vi "Begin.vi"() -> (0 "error out":errorcluster)   [LabVIEW 2013]
doc: "Called before other user functions, this VI is expected to open initial I/O refnums, load in file data, and do all program initialization. Notice that the <B>error out</B> terminal is simply used for data flow. Wiring it to other structures or subVIs ensures that this VI runs first."
uses:
  <vilib>/Rock Robotics/WPI/DriverStation/WPI_DriverStationRobotMode2.ctl
  <vilib>/Rock Robotics/WPI/Joystick/WPI_JoystickDeviceEnum.ctl
  <vilib>/Rock Robotics/SystemInterfaces/DIO/FPGA_DIORelayChannel.ctl
  <vilib>/Rock Robotics/SystemInterfaces/DIO/FPGA_DIOChannel.ctl
  <vilib>/Rock Robotics/SystemInterfaces/Typedef/FPGA_TypedefDigitalModule.ctl
  <vilib>/Rock Robotics/WPI/Solenoid/WPI_SolenoidChannel.ctl
  <vilib>/Rock Robotics/SystemInterfaces/DIO/FPGA_DIOPWMChannel.ctl
  <vilib>/Rock Robotics/WPI/SafetyOutput/WPI_SafetyOutputConfigMenu.ctl
  TankDriveAction.ctl
  PnuematicMode.ctl
  <vilib>/Rock Robotics/WPI/Camera/WPI_CameraWhite Balance Values.ctl
  <vilib>/Rock Robotics/WPI/Camera/WPI_CameraExposure Values.ctl
  <vilib>/Rock Robotics/WPI/Camera/WPI_CameraFrameRate.ctl
  <vilib>/Rock Robotics/WPI/Camera/WPI_CameraImageSize.ctl
  OccurrenceAction.ctl
  NotifierAction.ctl
  Example_Code/Gyro/Read Angle Mode.ctl
  <vilib>/Rock Robotics/SystemInterfaces/Typedef/FPGA_TypedefAnalogModuleForGyro.ctl
  <vilib>/Rock Robotics/SystemInterfaces/AI/FPGA_AIGyroChannel.ctl
  Robot Global Data.vi
  <vilib>/Rock Robotics/WPI/Solenoid/WPI_SolenoidOpenSingle.vi
  <vilib>/Rock Robotics/WPI/RobotDrive/WPI_RobotDriveOpen4MotorWithTalon.vi
  ErrorTest/OutputError.vi
  <vilib>/Rock Robotics/WPI/Compressor/WPI_CompressorGetSetRefNum.vi
  <vilib>/Rock Robotics/WPI/Counter/WPI_CounterDigitalInputToDigitalSource.vi
  <vilib>/Rock Robotics/WPI/Encoder/WPI_EncoderType.ctl
panel:
  in  "Gain (VoltsPerDegree/Second)":dbl=0.007
  in  "Version":string="1.3.1"
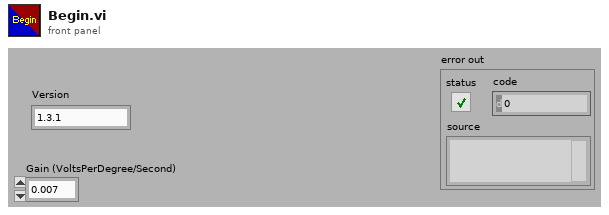
[diagram p1: front panel]
types:
  T1 = typedef "FPGA_AIGyroChannel.ctl" = enum8{"AI 1", "AI 2", "Invalid"}
  T2 = typedef "FPGA_TypedefAnalogModuleForGyro.ctl" = enum16{"Analog Module 1"}
  T3 = typedef "Read Angle Mode.ctl" = enum16{"Init", "ReadAngle", "Disable"}
  T4 = typedef "NotifierAction.ctl" = enum16{"Init", "Get"}
  T5 = typedef "OccurrenceAction.ctl" = enum16{"Init", "Get", "Set"}
  T6 = typedef "WPI_CameraImageSize.ctl" = enum16{"640x480", "320x240", "160x120"}
  T7 = typedef "WPI_CameraFrameRate.ctl" = u32
  T8 = typedef "WPI_CameraExposure Values.ctl" = enum16{"Auto", "Flicker-free 50 Hz", "Flicker-free 60 Hz", "Hold current"}
  T9 = typedef "WPI_CameraWhite Balance Values.ctl" = enum16{"Auto", "Fixed indoor", "Fixed outdoor 1", "Fixed outdoor 2", "Fixed fluorescent 1", "Fixed fluorescent 2", "Hold current"}
  T10 = typedef "PnuematicMode.ctl" = enum16{"Init", "SetState", "Disable"}
  T11 = typedef "WPI_SolenoidChannel.ctl" = enum8{"Solenoid 1", "Solenoid 2", "Solenoid 3", "Solenoid 4", "Solenoid 5", "Solenoid 6", "Solenoid 7", "Solenoid 8", "Invalid"}
  T12 = typedef "FPGA_DIOPWMChannel.ctl" = enum8{"PWM 1", "PWM 2", "PWM 3", "PWM 4", "PWM 5", "PWM 6", "PWM 7", "PWM 8", "PWM 9", "PWM 10", "Invalid"}
  T13 = typedef "TankDriveAction.ctl" = enum16{"Init", "LinearDrive", "SetValue", "Disable"}
  T14 = typedef "WPI_SafetyOutputConfigMenu.ctl" = enum16{"Enable", "Disable"}
  T15 = typedef "FPGA_TypedefDigitalModule.ctl" = enum16{"Digital Module 1", "Digital Module 2"}
  T16 = typedef "FPGA_DIOChannel.ctl" = enum8{"DIO 1", "DIO 2", "DIO 3", "DIO 4", "DIO 5", "DIO 6", "DIO 7", "DIO 8", "DIO 9", "DIO 10", "DIO 11", "DIO 12", "DIO 13", "DIO 14", "Invalid"}
  T17 = typedef "FPGA_DIORelayChannel.ctl" = enum8{"Relay 1", "Relay 2", "Relay 3", "Relay 4", "Relay 5", "Relay 6", "Relay 7", "Relay 8", "Invalid"}
  T18 = typedef "WPI_JoystickDeviceEnum.ctl" = enum16{"USB 1", "USB 2", "USB 3", "USB 4", "Kinect 1", "Kinect 2"}
  T19 = typedef "WPI_DriverStationRobotMode2.ctl" = enum16{"Autonomous Disabled", "Autonomous Enabled", "Teleop Disabled", "Teleop Enabled", "Timeout", "Finish", "Test Disabled", "Test Enabled"}
  T20 = typedef "WPI_EncoderType.ctl" = enum16{"1x", "2x", "4x"}
  T21 = typedef "WPI_DigitalInputDevRef.ctl" = cluster{"DevStatus":errorcluster, "DIO Channel":T16, "Digital Module":T15}
  T22 = typedef "FPGA_CounterEncoderSourceConvertionLVSourceType.ctl" = cluster{"DevStatus":errorcluster, "AnalogTriggerMode?":bool, "DigitalMode":cluster{"Digital Module":T15, "DIO Channel":T23}, "AnalogTriggerMode":cluster{"AnalogTriggerIndex":T24, "OutputType":T25}}
  T23 = typedef "FPGA_DIODigitalSourceChannel.ctl" = enum8{"DIO 1", "DIO 2", "DIO 3", "DIO 4", "DIO 5", "DIO 6", "DIO 7", "DIO 8", "DIO 9", "DIO 10", "DIO 11", "DIO 12", "DIO 13", "DIO 14", "Disabled"}
  T24 = typedef "FPGA_AnalogTriggerIndex.ctl" = enum8{"Trig 0", "Trig 1", "Trig 2", "Trig 3", "Trig 4", "Trig 5", "Trig 6", "Trig 7", "Invalid"}
  T25 = typedef "FPGA_AnalogTriggerOutType.ctl" = enum16{"InWindow", "TriggerState", "Rising", "Falling"}
  T26 = typedef "WPI_EncoderDevRef.ctl" = cluster{"DevStatus":errorcluster, "EncoderIndex":T27, "CounterIndex":T28, "DistancePerCount":dbl, "Decoding Type":T20}
  T27 = typedef "FPGA_EncoderIdx.ctl" = enum8{"Enc 0", "Enc 1", "Enc 2", "Enc 3", "Invalid"}
  T28 = typedef "FPGA_CounterCtrSystemIndex.ctl" = enum8{"Ctr 0", "Ctr 1", "Ctr 2", "Ctr 3", "Ctr 4", "Ctr 5", "Ctr 6", "Ctr 7", "Invalid"}
  T29 = typedef "WPI_SolenoidDevRef.ctl" = cluster{"DevStatus":errorcluster, "Solenoid Module":T30, "Forward Solenoid Channel":T11, "Reverse Solenoid Channel":T11}
  T30 = typedef "FPGA_TypedefSolenoidModule.ctl" = enum16{"Solenoid Module 1", "Solenoid Module 2"}
  T31 = typedef "WPI_RobotDriveDevRef.ctl" = cluster{"DevStatus":errorcluster, "Motors[]":T32[], "Square Inputs":bool, "Max Output":dbl, "Isochronous":bool}
  T32 = typedef "WPI_MotorControlDeviceRef.ctl" = cluster{"DeviceStatus":errorcluster, "Type":enum16{"PWM", "CAN"}, "PWM":cluster{"Digital Module":T15, "PWM Channel":T12, "DeadBand":T33}, "CAN":cluster{"Device Number":u8, "Control Mode":T34, "Semaphore":T35, "Max Vout":dbl}, "Invert":bool, "TransformRef":T36, "InvTransformRef":T36}
  T33 = typedef "WPI_PWMDeadband.ctl" = cluster{"Name":string, "maxPositivePwm":i32, "minPositivePwm":i32, "centerPwm":i32, "maxNegativePwm":i32, "minNegativePwm":i32, "angularRange":u16}
  T34 = typedef "WPI_CANJaguar_ControlMode.ctl" = enum8{"Percent VBus", "Current", "Speed", "Position", "Voltage"}
  T35 = typedef "Semaphore RefNum" = refnum<k1>
  T36 = typedef "WPI_PWMTransform_ConPane.ctl" = refnum<vi>
  T37 = typedef "WPI_CameraDevRef.ctl" = cluster{"Camera Address":string, "CameraStatus":errorcluster, "Acquire Image Notifier":refnum<notifier>}
  T38 = typedef "WPI_JoystickDevRef.ctl" = cluster{"Device":T18}
  T39 = typedef "WPI_CompressorDevRef.ctl" = cluster{"DevStatus":errorcluster, "DigitalInputDevRef":T21, "RelayDevRef":T40}
  T40 = typedef "WPI_RelayDevRef.ctl" = cluster{"DevStatus":errorcluster, "Relay Channel":T17, "Digital Module":T15, "Relay Direction":T41}
  T41 = typedef "WPI_RelayDirection.ctl" = enum16{"Both directions", "Forward only", "Reverse only"}
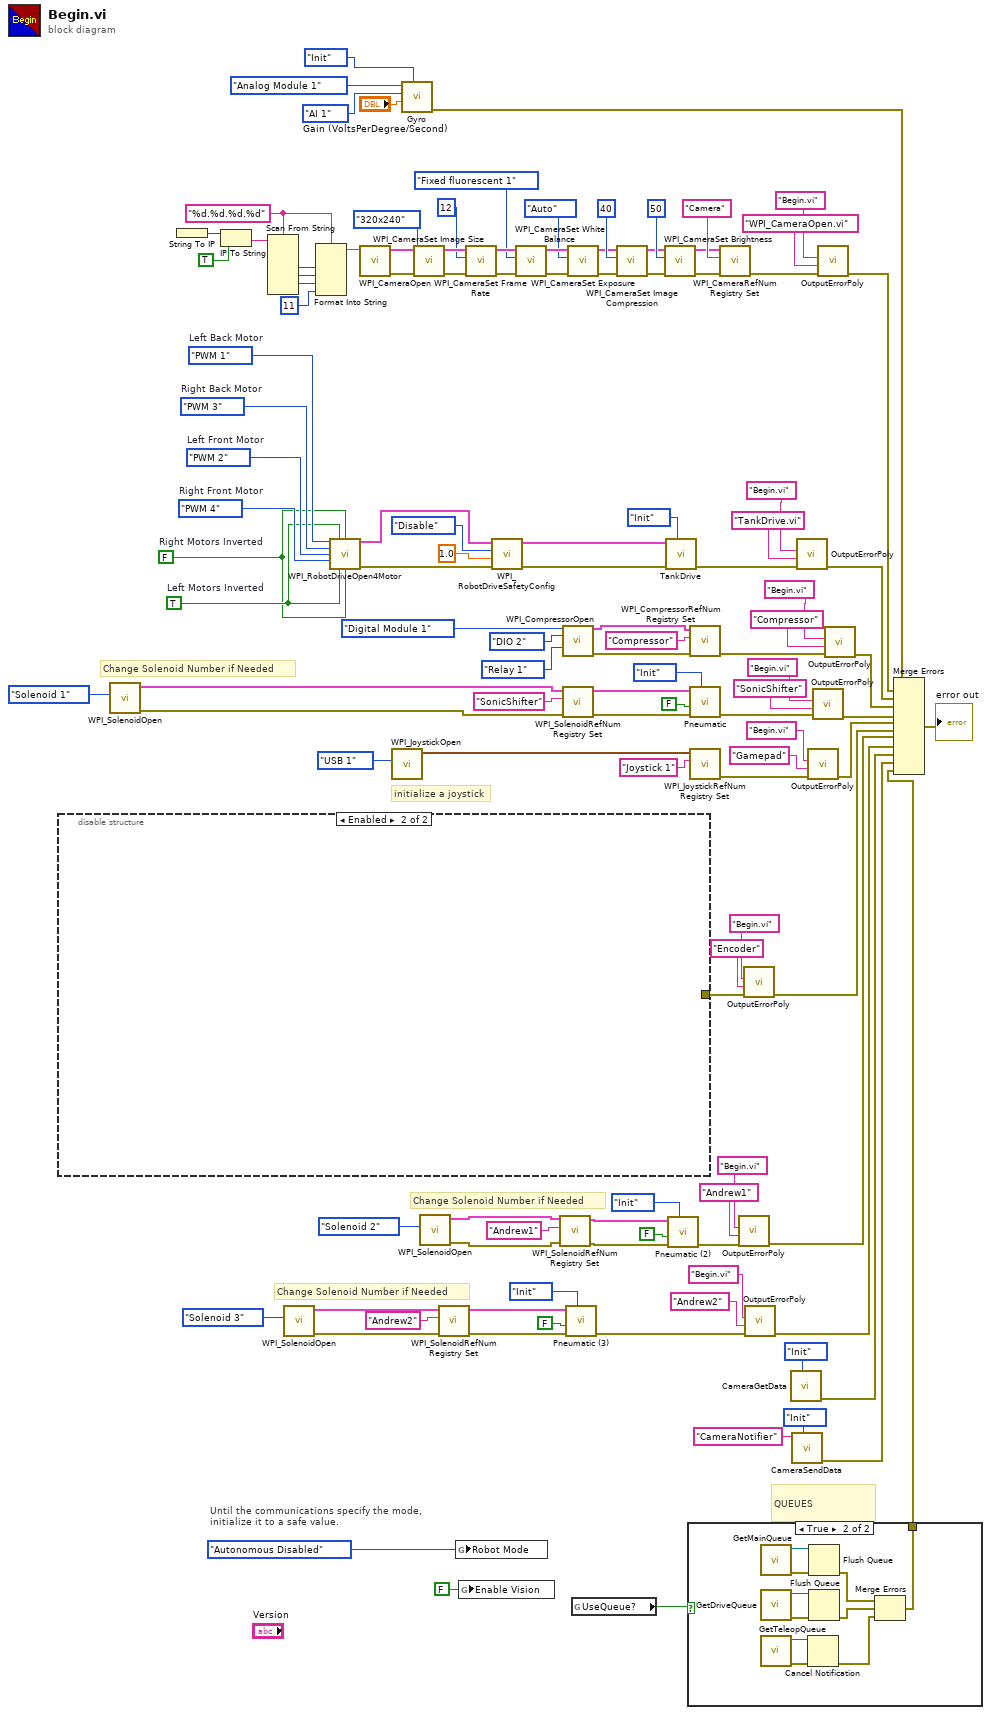
[diagram p0: block diagram]
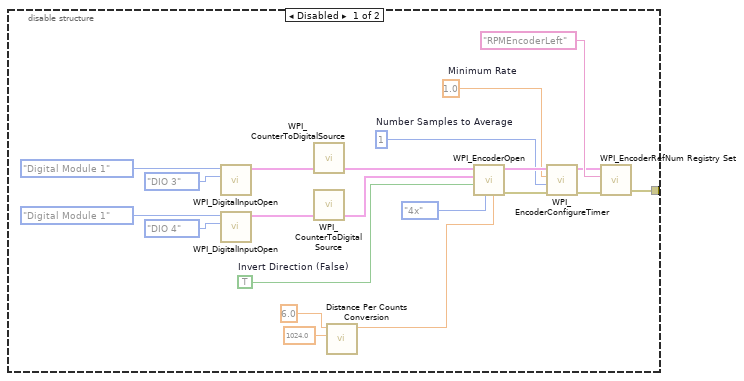
[diagram p3: hidden frame]
diagram:
  w51 = "%d.%d.%d.%d" ("format string")
  w103 = FPGA_DIOPWMChannel."PWM 4"  # Right Front Motor
  w104 = FPGA_DIOPWMChannel."PWM 2"  # Left Front Motor
  w109 = FPGA_DIOPWMChannel."PWM 3"  # Right Back Motor
  w110 = FPGA_DIOPWMChannel."PWM 1"  # Left Back Motor
  w101 = FALSE  # Right Motors Inverted
  w102 = TRUE  # Left Motors Inverted
  # "QUEUES"
  # "Change Solenoid Number if Needed"
  # "Change Solenoid Number if Needed"
  # "Change Solenoid Number if Needed"
  # "initialize a joystick"
  # "Until the communications specify the mode,\ninitialize it to a safe value."
  n1 = disable-structure shown="Enabled" {
    disable-tunnel: [w124 _] -> w33
    frame Disabled {
      w131 = TRUE  # Invert Direction (False)
      w133 = u8 1  # Number Samples to Average
      w134 = 1.0  # Minimum Rate
      n2 = call <vilib>:"WPI_DigitalInputOpen.vi"("DIO Channel"=FPGA_DIOChannel."DIO 3", "Digital Module (Module 1)"=FPGA_TypedefDigitalModule."Digital Module 1") -> ("DigitalInputDevRef"=w141:T21)  [unwired: 1 in, 8 out]
      n3 = call <vilib>:"WPI_DigitalInputOpen.vi"("DIO Channel"=FPGA_DIOChannel."DIO 4", "Digital Module (Module 1)"=FPGA_TypedefDigitalModule."Digital Module 1") -> ("DigitalInputDevRef"=w142:T21)  [unwired: 1 in, 8 out]
      n4 = call-poly <vilib>:"WPI_CounterToDigitalSource.vi"("DigitalInputDevRef"=w141) -> ("Digital Source"=w140:T22)  [unwired: 6 out]
      n5 = call-poly <vilib>:"WPI_CounterToDigitalSource.vi"("DigitalInputDevRef"=w142) -> ("Digital Source"=w143:T22)  [unwired: 6 out]
      n6 = call "Distance Per Counts Conversion.vi"("Counts Per Rev"=1024.0, "WheelDiameter"=6.0) -> ("Distance/Count"=w127:dbl)  [unwired: 9 in]
      n7 = call <vilib>:"WPI_EncoderOpen.vi"("DistancePerCount"=w127, "Decoding Type"=WPI_EncoderType."4x", "Invert Direction (False)"=w131, "BSource"=w143, "ASource"=w140) -> ("error out"=w129:errorcluster, "EncoderDevRef"=w137:T26)  [unwired: 3 in, 2 out]
      n8 = call <vilib>:"WPI_EncoderConfigureTimer.vi"("error in (no error)"=w129, "Number Samples to Average"=w133, "Minimum Rate"=w134, "EncoderDevRef"=w137) -> ("error out"=w128:errorcluster, "EncoderDevRef"=w130:T26)  [unwired: 6 out]
      n9 = call <vilib>:"WPI_EncoderRefNum Registry Set.vi"("error in (no error)"=w128, "refnum name"="RPMEncoderLeft", "EncoderDevRef"=w130) -> ("error out"=w124:errorcluster)  [unwired: 7 in, 1 out]
    }
    frame Enabled {
    }
  }
  n10 = call-poly <vilib>:"WPI_SolenoidOpen.vi"("Solenoid Channel"=WPI_SolenoidChannel."Solenoid 1") -> ("error out"=w111:errorcluster, "SolenoidDevRef"=w113:T29)  [unwired: 9 in]
  n11 = String To IP() -> (0:w58:u32)  [unwired: 1 in]
  n12 = IP To String(1:TRUE ("dot notation? (F)"), 2:w58) -> (0:w56:string)
  n13 = Scan From String(format string=w51, input string=w56) -> (output 1=w55:i32, output 2=w54:i32, output 3=w53:i32)  [unwired: 7 in, 3 out]
  n14 = call-poly <vilib>:"WPI_SolenoidOpen.vi"("Solenoid Channel"=WPI_SolenoidChannel."Solenoid 3") -> ("error out"=w92:errorcluster, "SolenoidDevRef"=w93:T29)  [unwired: 9 in]
  n15 = Format Into String(format string=w51, w55, w54, w53, 11 ("Compression")) -> (resulting string=w50:string)  [unwired: 2 in, 1 out]
  n16 = call-poly <vilib>:"WPI_RobotDriveOpen4Motor.vi"("Rear Left Motor"=w110, "Rear Left Motor Inverted"=w102, "Rear Right Motor Inverted"=w101, "Rear Right Motor"=w109, "Front Left Motor"=w104, "Front Right Motor"=w103, "Front Left Motor Inverted"=w102, "Front Right Motor Inverted"=w101) -> ("RobotDriveDevRef"=w108:T31, "error out"=w107:errorcluster)  [unwired: 6 in]
  n17 = call <vilib>:"WPI_CameraOpen.vi"("Camera Address"=w50) -> ("error out"=w69:errorcluster, "CameraDevRef"=w70:T37)  [unwired: 1 in, 8 out]
  n18 = call <vilib>:"WPI_JoystickOpen.vi"("JoystickDevice"=WPI_JoystickDeviceEnum."USB 1") -> ("JoystickDevRef"=w121:T38)  [unwired: 10 in]
  n19 = call "Gyro.vi"("Enum"=Read_Angle_Mode."Init", "Gain (VoltsPerDegree/Second) 2"="Gain (VoltsPerDegree/Second)", "Channel 2"=FPGA_AIGyroChannel."AI 1", "Analog Module 2"=FPGA_TypedefAnalogModuleForGyro."Analog Module 1") -> ("error out"=w2:errorcluster)  [unwired: 6 in, 1 out]
  n20 = call <vilib>:"WPI_CameraSet Image Size.vi"("error in (no error)"=w69, "Image Size"=WPI_CameraImageSize."320x240", "CameraDevRef"=w70) -> ("error out"=w68:errorcluster, "CameraDevRef Out"=w71:T37)  [unwired: 7 out]
  n21 = call-poly <vilib>:"WPI_SolenoidOpen.vi"("Solenoid Channel"=WPI_SolenoidChannel."Solenoid 2") -> ("error out"=w95:errorcluster, "SolenoidDevRef"=w97:T29)  [unwired: 9 in]
  n22 = call <vilib>:"WPI_SolenoidRefNum Registry Set.vi"("error in (no error)"=w92, "refnum name"="Andrew2", "SolenoidDevRef"=w93) -> ("error out"=w84:errorcluster, "SolenoidDevRef"=w83:T29)  [unwired: 7 in]
  n23 = global write "Robot Global Data.vi" "Robot Mode"(WPI_DriverStationRobotMode2."Autonomous Disabled" ("Robot Mode")) -> ()
  n24 = global write "Robot Global Data.vi" "Enable Vision"(FALSE ("Enable Vision")) -> ()
  n25 = call <vilib>:"WPI_CameraSet Frame Rate.vi"("error in (no error)"=w68, "Frame Rate (fps)"=T7 12, "CameraDevRef"=w71) -> ("error out"=w67:errorcluster, "CameraDevRef Out"=w73:T37)  [unwired: 7 out]
  n26 = call <vilib>:"WPI_RobotDriveSafetyConfig.vi"("error in (no error)"=w107, "timeout (s)"=1.0, "mode"=WPI_SafetyOutputConfigMenu."Disable", "RobotDriveDevRef"=w108) -> ("error out"=w46:errorcluster, "RobotDriveDevRef"=w45:T31)  [unwired: 6 in]
  n27 = call <vilib>:"WPI_CameraSet White Balance.vi"("error in (no error)"=w67, "White Balance"=WPI_CameraWhite_Balance_Values."Fixed fluorescent 1", "CameraDevRef"=w73) -> ("error out"=w66:errorcluster, "CameraDevRef Out"=w72:T37)  [unwired: 7 out]
  n28 = call <vilib>:"WPI_SolenoidRefNum Registry Set.vi"("error in (no error)"=w95, "refnum name"="Andrew1", "SolenoidDevRef"=w97) -> ("error out"=w87:errorcluster, "SolenoidDevRef"=w88:T29)  [unwired: 7 in]
  n29 = call <vilib>:"WPI_CompressorOpen.vi"("Pressure Switch Digital Module (Module 1)"=FPGA_TypedefDigitalModule."Digital Module 1" ("Pressure Switch\nand Relay Module"), "Pressure Switch DIO Channel"=FPGA_DIOChannel."DIO 2" ("Pressure Switch Channel"), "Relay Channel"=FPGA_DIORelayChannel."Relay 1") -> ("CompressorDevRef"=w116:T39, "error out"=w100:errorcluster)  [unwired: 2 in, 9 out]
  n30 = call <vilib>:"WPI_SolenoidRefNum Registry Set.vi"("error in (no error)"=w111, "refnum name"="SonicShifter", "SolenoidDevRef"=w113) -> ("error out"=w90:errorcluster, "SolenoidDevRef"=w91:T29)  [unwired: 7 in]
  n31 = call "Pneumatic (3).vi"("Mode"=PnuematicMode."Init", "error in (no error)"=w84, "Default Position"=FALSE, "SolenoidDevRef"=w83) -> ("error out"=w29:errorcluster)  [unwired: 7 in]
  n32 = call <vilib>:"WPI_CameraSet Exposure.vi"("error in (no error)"=w66, "Exposure"=WPI_CameraExposure_Values."Auto", "CameraDevRef"=w72) -> ("error out"=w65:errorcluster, "CameraDevRef Out"=w75:T37)  [unwired: 7 out]
  n33 = global read "Robot Global Data.vi" "UseQueue?"() -> (w7:bool)
  n34 = call <vilib>:"WPI_CameraSet Image Compression.vi"("error in (no error)"=w65, "Compression"=40, "CameraDevRef"=w75) -> ("error out"=w64:errorcluster, "CameraDevRef Out"=w74:T37)  [unwired: 7 out]
  n35 = call <vilib>:"WPI_CameraSet Brightness.vi"("error in (no error)"=w64, "Brightness"=50, "CameraDevRef"=w74) -> ("error out"=w62:errorcluster, "CameraDevRef Out"=w63:T37)  [unwired: 7 out]
  n36 = call "TankDrive.vi"("DriveAction"=TankDriveAction."Init" ("Enum"), "error in (no error)"=w46, "RobotDriveDevRef"=w45) -> ("error out"=w41:errorcluster)  [unwired: 8 in]
  n37 = call "Pneumatic (2).vi"("Mode"=PnuematicMode."Init", "error in (no error)"=w87, "Default Position"=FALSE, "SolenoidDevRef"=w88) -> ("error out"=w31:errorcluster)  [unwired: 7 in]
  n38 = case shown="True" w7 {
    tunnel: [_ w145] -> w8
    frame False {
    }
    frame True {
      n39 = call "GetMainQueue.vi"() -> ("error out"=w154:errorcluster, "queue out"=w153:refnum<queue>)  [unwired: 10 in]
      n40 = call "GetDriveQueue.vi"() -> ("error out"=w152:errorcluster, "queue out"=w151:refnum<queue>)  [unwired: 10 in]
      n41 = call "GetTeleopQueue.vi"() -> ("error out"=w150:errorcluster, "notifier out"=w149:refnum<notifier>)  [unwired: 10 in]
      n42 = Cancel Notification(0:w149, 3:w150) -> (11:w146:errorcluster)  [unwired: 2 out]
      n43 = Flush Queue(queue=w153, error in (no error)=w154) -> (error out=w148:errorcluster)  [unwired: 2 out]
      n44 = Flush Queue(queue=w151, error in (no error)=w152) -> (error out=w147:errorcluster)  [unwired: 2 out]
      n45 = Merge Errors(w148, w147, w146) -> (w145:errorcluster)
    }
  }
  n46 = call <vilib>:"WPI_CompressorRefNum Registry Set.vi"("error in (no error)"=w100, "refnum name"="Compressor", "CompressorDevRef"=w116) -> ("error out"=w39:errorcluster)  [unwired: 7 in, 1 out]
  n47 = call "Pneumatic.vi"("Mode"=PnuematicMode."Init", "error in (no error)"=w90, "Default Position"=FALSE, "SolenoidDevRef"=w91) -> ("error out"=w37:errorcluster)  [unwired: 7 in]
  n48 = call <vilib>:"WPI_JoystickRefNum Registry Set.vi"("refnum name"="Joystick 1", "JoystickDevRef"=w121) -> ("error out"=w35:errorcluster)  [unwired: 8 in, 1 out]
  n49 = call <vilib>:"WPI_CameraRefNum Registry Set.vi"("error in (no error)"=w62, "refnum name"="Camera", "CameraDevRef"=w63) -> ("error out"=w49:errorcluster)  [unwired: 8 out]
  n50 = call-poly "OutputErrorPoly.vi"("error in (no error)"=w31, "Causing VI"="Andrew1" ("Calling VI"), "Calling VI"="Begin.vi") -> ("error out"=w30:errorcluster)  [unwired: 8 in]
  n51 = call-poly "OutputErrorPoly.vi"("error in (no error)"=w33, "Causing VI"="Encoder" ("Calling VI"), "Calling VI"="Begin.vi") -> ("error out"=w32:errorcluster)  [unwired: 8 in]
  n52 = call-poly "OutputErrorPoly.vi"("error in (no error)"=w29, "Causing VI"="Andrew2" ("Calling VI"), "Calling VI"="Begin.vi") -> ("error out"=w28:errorcluster)  [unwired: 8 in]
  n53 = call "CameraGetData.vi"("Action"=OccurrenceAction."Init") -> ("error out"=w12:errorcluster)  [unwired: 9 in, 1 out]
  n54 = call "CameraSendData.vi"("Action"=NotifierAction."Init", "name (unnamed)"="CameraNotifier") -> ("error out"=w9:errorcluster)  [unwired: 8 in, 1 out]
  n55 = call-poly "OutputErrorPoly.vi"("error in (no error)"=w41, "Causing VI"="TankDrive.vi" ("Calling VI"), "Calling VI"="Begin.vi") -> ("error out"=w40:errorcluster)  [unwired: 8 in]
  n56 = call-poly "OutputErrorPoly.vi"("error in (no error)"=w35, "Causing VI"="Gamepad" ("Calling VI"), "Calling VI"="Begin.vi") -> ("error out"=w34:errorcluster)  [unwired: 8 in]
  n57 = call-poly "OutputErrorPoly.vi"("error in (no error)"=w37, "Causing VI"="SonicShifter" ("Calling VI"), "Calling VI"="Begin.vi") -> ("error out"=w36:errorcluster)  [unwired: 8 in]
  n58 = call-poly "OutputErrorPoly.vi"("error in (no error)"=w49, "Causing VI"="WPI_CameraOpen.vi" ("Calling VI"), "Calling VI"="Begin.vi") -> ("error out"=w1:errorcluster)  [unwired: 8 in]
  n59 = call-poly "OutputErrorPoly.vi"("error in (no error)"=w39, "Causing VI"="Compressor" ("Calling VI"), "Calling VI"="Begin.vi") -> ("error out"=w38:errorcluster)  [unwired: 8 in]
  n60 = Merge Errors(w2, w1, w40, w38, w36, w34, w32, w30, w28, w12, w9, w8) -> (→"error out":errorcluster)
